vi "90D_Pulse_CommandSTR_gen.vi"(11 "90 Degree Pulse Sequence":T2={"Delay Settings"={"Delay d1"=10.0, "Delay d2"=0.0, "d1 Unit"=0, "d2 Unit"=0}, "Preliminary Settings"={"Nº of Scans (ns)"=3, "Pulse Frequency"=10000000.0}, "Pulse Settings"={"Duration Signal P1"=20.0, "Power Level"=1023, "Phase"=90, "P1 Units"=0}, "Acquisition Settings"={"Number Samples"=2000, "Time Between Points"=0.0, "Unit"=0}} {"Acquisition Settings"."Unit" items=["us", "ms"]; "Acquisition Settings"."Time Between Points" min=0.0 step=1.0; "Acquisition Settings"."Number Samples" step=1; "Pulse Settings"."P1 Units" items=["us", "ms"]; "Pulse Settings"."Phase" max=270 step=90; "Pulse Settings"."Power Level" max=1023 step=1; "Pulse Settings"."Duration Signal P1" min=0.0 step=1.0 format="%#_4g"; "Preliminary Settings"."Pulse Frequency" min=1.0 max=200000000.0 step=1000000.0 format="%^#_6e"; "Preliminary Settings"."Nº of Scans (ns)" step=1; "Delay Settings"."d2 Unit" items=["us", "ms"]; "Delay Settings"."d1 Unit" items=["us", "ms"]; "Delay Settings"."Delay d2" min=0.0 step=1.0 format="%#_4g"; "Delay Settings"."Delay d1" min=0.0 step=1.0 format="%#_4g"}) -> (2 "90 Set Times":T1, 3 "CMD STR Array":string[](array[string]))   [LabVIEW 2011]
uses:
  Controls/Full_90 Degree Pulse Settings.ctl
  Controls/90D_Delay Settings.ctl
  Controls/90D_Preliminary Settings.ctl
  Controls/90D_Pulse Settings.ctl
  Controls/Acquisition Settings.ctl
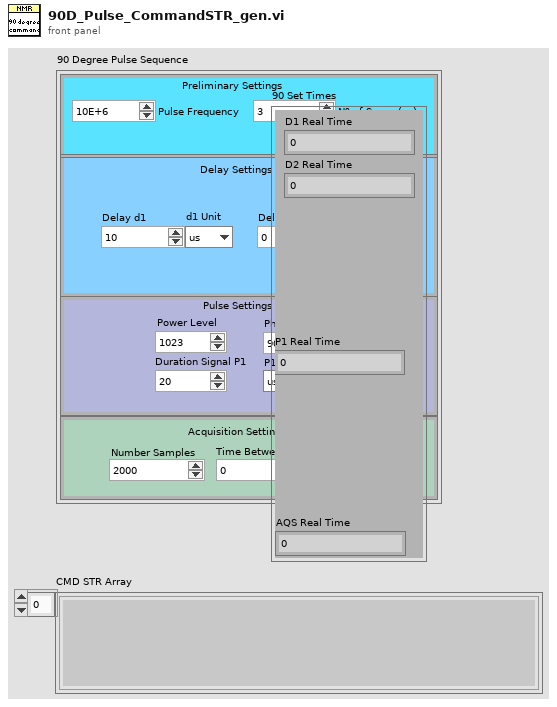
[diagram p1: front panel]
types:
  T1 = cluster{"D1 Real Time":ext, "D2 Real Time":ext, "P1 Real Time":ext, "AQS Real Time":ext}
  T2 = typedef "Full_90 Degree Pulse Settings.ctl" = cluster{"Delay Settings":T3, "Preliminary Settings":T4, "Pulse Settings":T5, "Acquisition Settings":T6}
  T3 = typedef "90D_Delay Settings.ctl" = cluster{"Delay d1":dbl, "Delay d2":dbl, "d1 Unit":u8, "d2 Unit":u8}
  T4 = typedef "90D_Preliminary Settings.ctl" = cluster{"Nº of Scans (ns)":u16, "Pulse Frequency":dbl}
  T5 = typedef "90D_Pulse Settings.ctl" = cluster{"Duration Signal P1":dbl, "Power Level":u16, "Phase":u16, "P1 Units":u8}
  T6 = typedef "Acquisition Settings.ctl" = cluster{"Number Samples":u16, "Time Between Points":dbl, "Unit":u8}
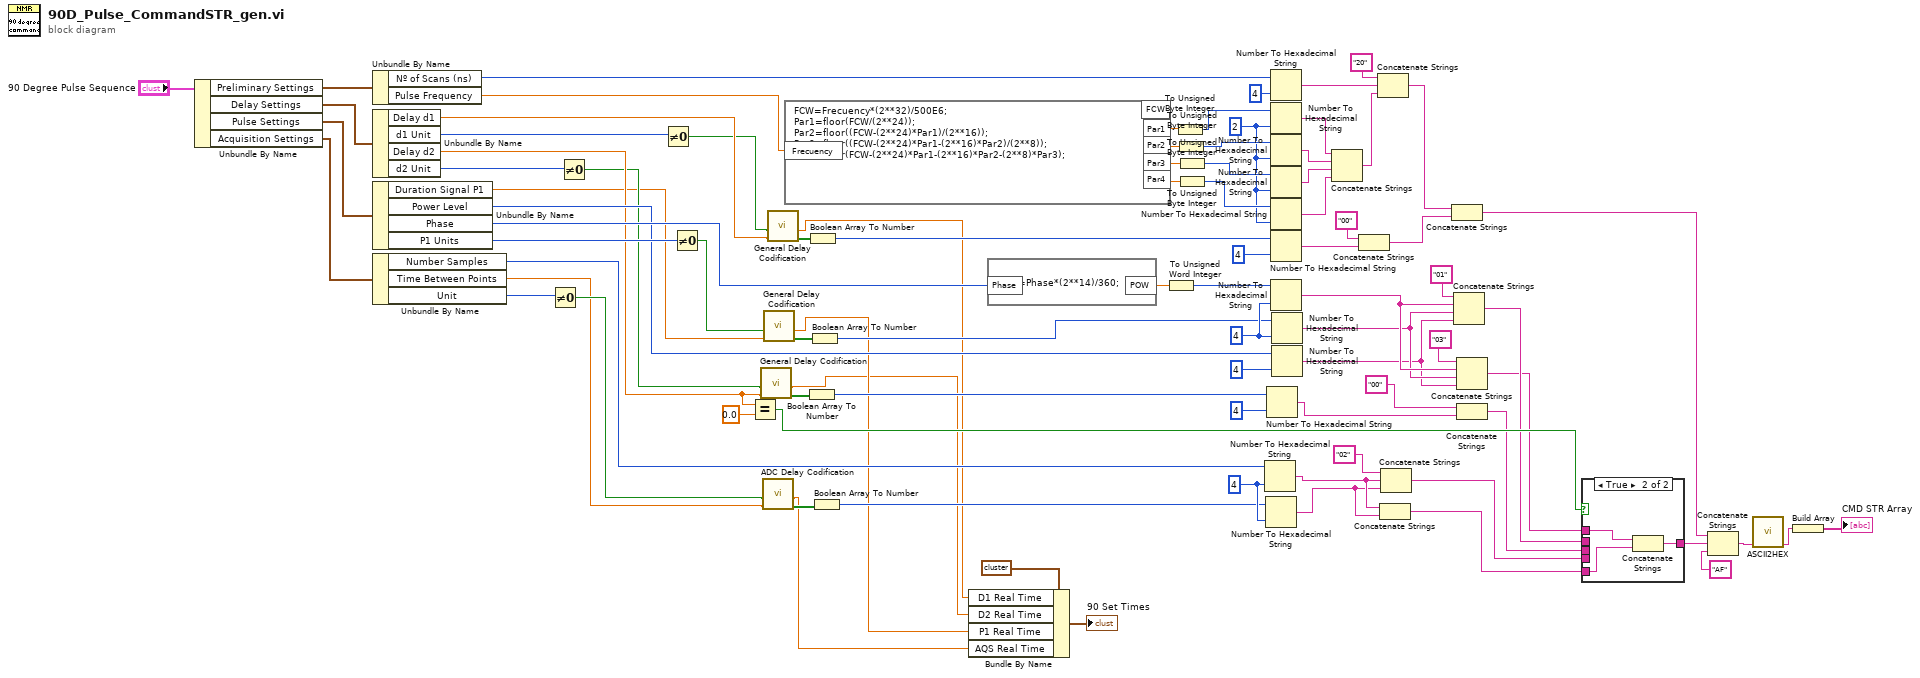
[diagram p0: block diagram]
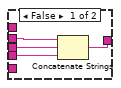
[diagram p2: hidden frame]
diagram:
  w56 = i16 2 ("width (-)")
  w77 = i16 4 ("width (-)")
  w86 = i16 4 ("width (-)")
  n1 = Unbundle By Name("90 Degree Pulse Sequence") -> ("Preliminary Settings"=w33:T4, "Delay Settings"=w32:T3, "Pulse Settings"=w30:T5, "Acquisition Settings"=w31:T6)
  n2 = Unbundle By Name(w33) -> ("Nº of Scans (ns)"=w29:u16, "Pulse Frequency"=w28:dbl)
  n3 = Unbundle By Name(w32) -> ("Delay d1"=w19:dbl, "d1 Unit"=w26:u8, "Delay d2"=w13:dbl, "d2 Unit"=w23:u8)
  n4 = Unbundle By Name(w30) -> ("Duration Signal P1"=w11:dbl, "Power Level"=w24:u16, "Phase"=w27:u16, "P1 Units"=w25:u8)
  n5 = Unbundle By Name(w31) -> ("Number Samples"=w22:u16, "Time Between Points"=w15:dbl, "Unit"=w21:u8)
  n6 = Not Equal To 0?(x=w21) -> (x != 0?=w16:bool)
  n7 = Not Equal To 0?(x=w23) -> (x != 0?=w12:bool)
  n8 = Not Equal To 0?(x=w26) -> (x != 0?=w18:bool)
  n9 = Not Equal To 0?(x=w25) -> (x != 0?=w10:bool)
  n10 = Equal?(x=w13, y=0.0) -> (x = y?=w49:bool)
  n11 = call "General Delay Codification.vi"("Delay"=w13, "ms/us Delay"=w12) -> ("Final array"=w14:bool[], "Real Time"=w2:ext)  [unwired: 8 in]
  n12 = call "ADC Delay Codification.vi"("Delay"=w15, "ms/us Delay"=w16) -> ("Final array"=w17:bool[], "Real Time"=w1:ext)  [unwired: 8 in]
  n13 = call "General Delay Codification.vi"("Delay"=w11, "ms/us Delay"=w10) -> ("Final array"=w9:bool[], "Real Time"=w3:ext)  [unwired: 8 in]
  n14 = call "General Delay Codification.vi"("Delay"=w19, "ms/us Delay"=w18) -> ("Final array"=w20:bool[], "Real Time"=w4:ext)  [unwired: 8 in]
  n15 = formula code="FCW=Frecuency*(2**32)/500E6;\nPar1=floor(FCW/(2**24));\nPar2=floor((FCW-(2**24)*Par1)/(2**16));\nPar3=floor((FCW-(2**24)*Par1-(2**16)*Par2)/(2**8));\nPar4=floor(FCW-(2**24)*Par1-(2**16)*Par2-(2**8)*Par3);"("Frecuency"=w28) -> ("Par1"=w60:dbl, "Par2"=w59:dbl, "Par3"=w58:dbl, "Par4"=w57:dbl)  [unwired: 1 out]
  n16 = Boolean Array To Number(Boolean array=w14) -> (number=w68:u32)
  n17 = Boolean Array To Number(Boolean array=w20) -> (number=w70:u32)
  n18 = Boolean Array To Number(Boolean array=w9) -> (number=w69:u32)
  n19 = Boolean Array To Number(Boolean array=w17) -> (number=w67:u32)
  n20 = Bundle By Name(cluster=T1 {"D1 Real Time"=0.0, "D2 Real Time"=0.0, "P1 Real Time"=0.0, "AQS Real Time"=0.0} ("Set Times"), "D1 Real Time"=w4, "D2 Real Time"=w2, "P1 Real Time"=w3, "AQS Real Time"=w1) -> (→"90 Set Times":T1)
  n21 = formula code="POW=Phase*(2**14)/360;"("Phase"=w27) -> ("POW"=w66:dbl)
  n22 = To Unsigned Word Integer(number=w66) -> (unsigned 16bit integer=w65:u16)
  n23 = To Unsigned Byte Integer(number=w60) -> (unsigned 8bit integer=w64:u8)
  n24 = To Unsigned Byte Integer(number=w59) -> (unsigned 8bit integer=w63:u8)
  n25 = To Unsigned Byte Integer(number=w58) -> (unsigned 8bit integer=w62:u8)
  n26 = To Unsigned Byte Integer(number=w57) -> (unsigned 8bit integer=w61:u8)
  n27 = Number To Hexadecimal String(1:w77, 2:w22) -> (0:w39:string)
  n28 = Number To Hexadecimal String(1:w77, 2:w67) -> (0:w38:string)
  n29 = Number To Hexadecimal String(1:i16 4 ("width (-)"), 2:w68) -> (0:w79:string)
  n30 = Number To Hexadecimal String(1:i16 4 ("width (-)"), 2:w29) -> (0:w75:string)
  n31 = Number To Hexadecimal String(1:w56, 2:w64) -> (0:w55:string)
  n32 = Number To Hexadecimal String(1:w56, 2:w63) -> (0:w54:string)
  n33 = Number To Hexadecimal String(1:w56, 2:w62) -> (0:w53:string)
  n34 = Number To Hexadecimal String(1:w56, 2:w61) -> (0:w52:string)
  n35 = Number To Hexadecimal String(1:i16 4 ("width (-)"), 2:w70) -> (0:w83:string)
  n36 = Number To Hexadecimal String(1:w86, 2:w65) -> (0:w44:string)
  n37 = Number To Hexadecimal String(1:w86, 2:w69) -> (0:w43:string)
  n38 = Number To Hexadecimal String(1:i16 4 ("width (-)"), 2:w24) -> (0:w42:string)
  n39 = Concatenate Strings(w55, w54, w53, w52) -> (w51:string)
  n40 = Concatenate Strings("00" ("string"), w83) -> (w72:string)
  n41 = Concatenate Strings("20" ("string"), w75, w51) -> (w73:string)
  n42 = Concatenate Strings(w39, w38) -> (w37:string)
  n43 = Concatenate Strings("02" ("string"), w39, w38) -> (w45:string)
  n44 = Concatenate Strings(w73, w72) -> (w71:string)
  n45 = Concatenate Strings("01" ("string"), w44, w43, w42) -> (w47:string)
  n46 = Concatenate Strings("03" ("string"), w44, w43, w42) -> (w40:string)
  n47 = Concatenate Strings("00" ("string"), w79) -> (w48:string)
  n48 = case shown="True" w49 {
    tunnel: w48 -> [w90 _]
    tunnel: w47 -> [w91 _]
    tunnel: [w88 w92] -> w46
    tunnel: w45 -> [w89 _]
    tunnel: w40 -> [_ w94]
    tunnel: w37 -> [_ w93]
    frame False {
      n49 = Concatenate Strings(w91, w90, w89) -> (w88:string)
    }
    frame True {
      n50 = Concatenate Strings(w94, w93) -> (w92:string)
    }
  }
  n51 = Concatenate Strings(w71, w46, "AF" ("string")) -> (w35:string)
  n52 = call "ASCII2HEX.vi"("String (Normal Display)"=w35) -> ("Result string (Hex Display)"=w8:string)  [unwired: 10 in]
  n53 = Build Array(w8) -> (→"CMD STR Array":string[])
